vi "frequency analysis.vi"(9 "Pattern frequency (Hz)":dbl, 10 "Frecuencia de muestreo (Hz)":dbl, 11 "Calibration":T1) -> (0 "Frecuencias validas":bool[](array[boolean]), 1 "Magnitude*df":dbl[](array[numeric]), 2 "mean":dbl format="%0.2f", 3 "output calibration":T1)   [LabVIEW 2015]
uses:
  controls/Calibration Data.ctl
  <vilib>/measure/maspectr.llb/FFT Spectrum (Mag-Phase) for 1 Chan.vi
  <vilib>/measure/NI_MAPro.lvlib
  <vilib>/Analysis/NI_AALBase.lvlib
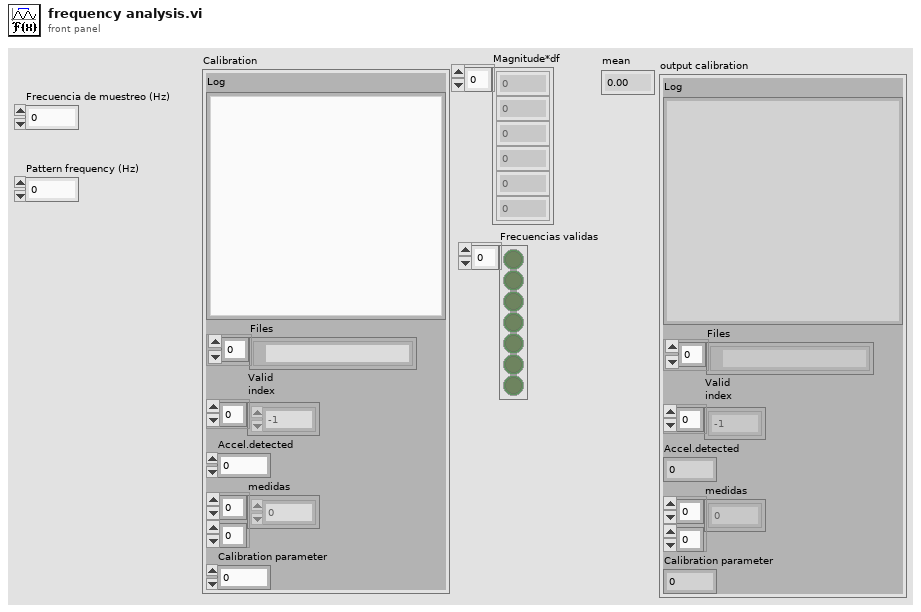
[diagram p1: front panel]
types:
  T1 = typedef "Calibration Data.ctl" = cluster{"Log":string, "Files":path[], "Valid\nindex":i32[], "Accel.detected":i32, "medidas":sgl[][], "Calibration parameter":dbl}
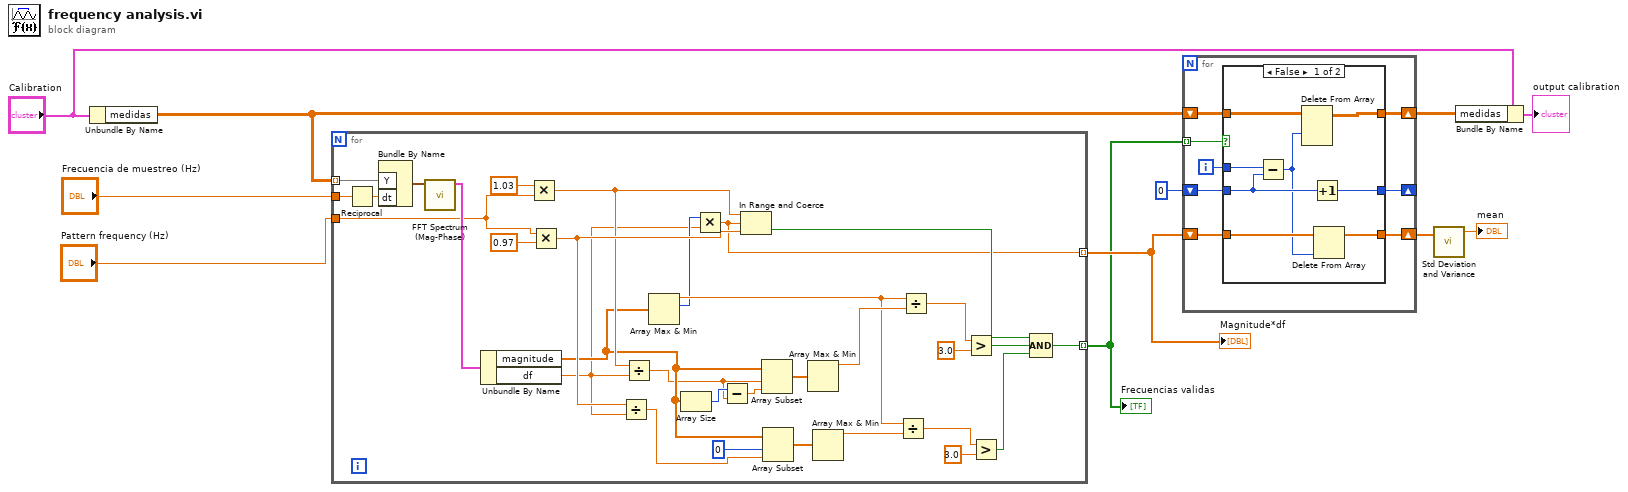
[diagram p0: block diagram]
diagram:
  n1 = Unbundle By Name("Calibration") -> ("medidas"=w11:sgl[][])
  n2 = for {
    tunnel: w11 -> [w42] mode=indexing
    tunnel: "Frecuencia de muestreo (Hz)" -> [w41]
    tunnel: "Pattern frequency (Hz)" -> [w37]
    tunnel: [w18] -> w3 mode=indexing
    tunnel: [w13] -> w7 mode=indexing
    n3 = Reciprocal(x=w41) -> (1/x=w43:dbl)
    n4 = Bundle By Name("Y"=w42, "dt"=w43) -> (w40:waveform(sgl))  [unwired: 1 in]
    n5 = call-poly <vilib>:"FFT Spectrum (Mag-Phase).vi"("time signal"=w40) -> ("magnitude"=w39:cluster{"f0":dbl, "df":dbl, "magnitude":dbl[]})  [unwired: 6 in, 4 out]
    n6 = Unbundle By Name(w39) -> ("magnitude"=w31:dbl[], "df"=w12:dbl)
    n7 = Multiply(x=1.03, y=w37) -> (x*y=w34:dbl)
    n8 = Multiply(x=w37, y=0.97 ("x")) -> (x*y=w35:dbl)
    n9 = Divide(x=w35, y=w12) -> (x/y=w32:dbl)
    n10 = Divide(x=w34, y=w12) -> (x/y=w29:dbl)
    n11 = Array Max & Min(array=w31) -> (max value=w24:dbl, max index (indices)=w14:i32)  [unwired: 2 out]
    n12 = Array Size(array=w31) -> (size(s)=w30:i32)
    n13 = Multiply(x=w14, y=w12) -> (x*y=w13:dbl)
    n14 = Subtract(x=w30, y=w29) -> (x-y=w28:dbl)
    n15 = In Range and Coerce(upper limit=w34, x=w13, lower limit=w35) -> (In Range?=w17:bool)  [unwired: 1 out]
    n16 = Array Subset(array=w31, index=w29, length=w28) -> (w27:dbl[])
    n17 = Array Subset(array=w31, index=0, length=w32) -> (w26:dbl[])
    n18 = Array Max & Min(array=w27) -> (max value=w25:dbl)  [unwired: 3 out]
    n19 = Array Max & Min(array=w26) -> (max value=w23:dbl)  [unwired: 3 out]
    n20 = Divide(x=w24, y=w23) -> (x/y=w21:dbl)
    n21 = Divide(x=w24, y=w25) -> (x/y=w22:dbl)
    n22 = Greater?(x=w22, y=3.0) -> (0:w16:bool)
    n23 = Greater?(x=w21, y=3.0) -> (0:w15:bool)
    n24 = Compound Arithmetic op=AND(w17, w16, w15) -> (w18:bool)
  }
  "Magnitude*df" <- w7
  "Frecuencias validas" <- w3
  n25 = for {
    shift-right: [w50] -> w5
    shift-left: w11 -> [w51]
    tunnel: w3 -> [w49] mode=indexing
    shift-right: [w46] -> _
    shift-left: 0 ("index of element") -> [w47]
    shift-right: [w44] -> w10
    shift-left: w7 -> [w45]
    i -> [w48]
    n26 = case shown="False" w49 {
      tunnel: w51 -> [w59 w62]
      tunnel: [w58 w62] -> w50
      tunnel: w48 -> [w57 _]
      tunnel: w47 -> [w56 w61]
      tunnel: [w55 w61] -> w46
      tunnel: w45 -> [w54 w60]
      tunnel: [w52 w60] -> w44
      frame False {
        n27 = Subtract(x=w57, y=w56) -> (x-y=w53:i32)
        n28 = Delete From Array(array=w59, index (row)=w53) -> (array with subset deleted=w58:sgl[][])  [unwired: 2 in, 1 out]
        n29 = Increment(x=w56) -> (x+1=w55:i32)
        n30 = Delete From Array(array=w54, index=w53) -> (array with subset deleted=w52:dbl[])  [unwired: 1 in, 1 out]
      }
      frame True {
      }
    }
  }
  n31 = call <vilib>:"Std Deviation and Variance.vi"("X"=w10) -> ("mean"=→"mean":dbl)  [unwired: 1 in, 2 out]
  n32 = Bundle By Name(cluster="Calibration", "medidas"=w5) -> (→"output calibration":T1)
